vi "Sleep.vi"(8 "error in (no error)":errorcluster, 11 "CIFCorePlugin in":refnum<class "CIFCorePlugin.lvclass">) -> (0 "error out":errorcluster, 2 "Housekeep only":bool, 3 "CIFCorePlugin out":refnum<class "CIFCorePlugin.lvclass">)   [LabVIEW 2021, in "CIFCorePlugin.lvclass"]
uses:
  CIFCorePlugin.lvclass
  CIFCorePlugin.lvclass/CIFCorePlugin.ctl
  Common/Typedef/Errors.ctl
  Accessors/Read Sleep Limits (ns).vi
  Accessors/Timestamps/Write Target Wake TS.vi
  Accessors/Timestamps/Read Running TS.vi
  Accessors/Read Running Internal Data.vi
  Accessors/Read Timing Override.vi
  Accessors/Read Common Config.vi
  <vilib>/CIF Foundation/CIF Utilities/Errors/Append Error Location.vi
  <vilib>/CIF Foundation/CIF Utilities/Time/System Time/LabVIEW Time to TAI Time.vi
  Common/CIFCoreCommon.lvlib
  <vilib>/CIF Foundation/CIF Utilities/Time/Time_CIF_U.lvlib
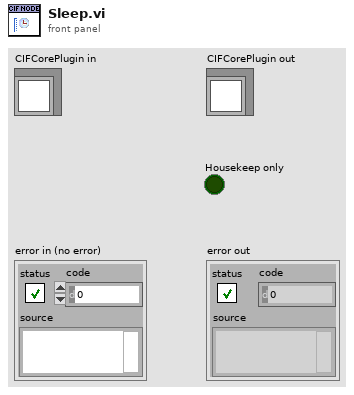
[diagram p1: front panel]
types:
  T1 = typedef "CIFCoreCommon.lvlib/Errors.ctl" = enum16{"Invalid Clock ID", "Long Sleep", "gRPC Server Not Found", "Config Parse", "Timestamp Wrap", "Delayed Execution", "Duplicate Channel", "Missing Channel", "Incorrect Type", "Flatten Error", "Unflatten Data", "Unique Name", "Plugin Not Found", "Plugin Type Not Found", "Plugin Version Not Found", "Manager Not Found", "Numerical Issue", "Time Jump", "Clock ID Match", "Channel Length", "Plugin Connection", "gRPC Server Connection", "PPL Name Match", "Build", "Config Log Parse", "Plugin Load"}
  T2 = typedef "CIFCoreCommon.lvlib/Timing Overrides.ctl" = cluster{"Override Timing":bool, "Skip Sleep":bool, "Period (s)":dbl}
  T3 = typedef "CIFCorePlugin.lvclass/Running Internal Data.ctl" = cluster{"Refresh":bool, "Iterations":i64, "Housekeep only":bool, "Configured period (ns)":i64, "Update channel OOB":bool}
  T4 = typedef "CIFCoreCommon.lvlib/Common Plugin Configuration.ctl" = cluster{"Period (s)":dbl, "Offset (us)":i32, "ClockID":u8, "Priority":i32, "Processor":i32}
  T5 = typedef "Time_CIF_U.lvlib/Future Time Event Limits.ctl" = cluster{"Maximum":i64, "Minimum":i64}
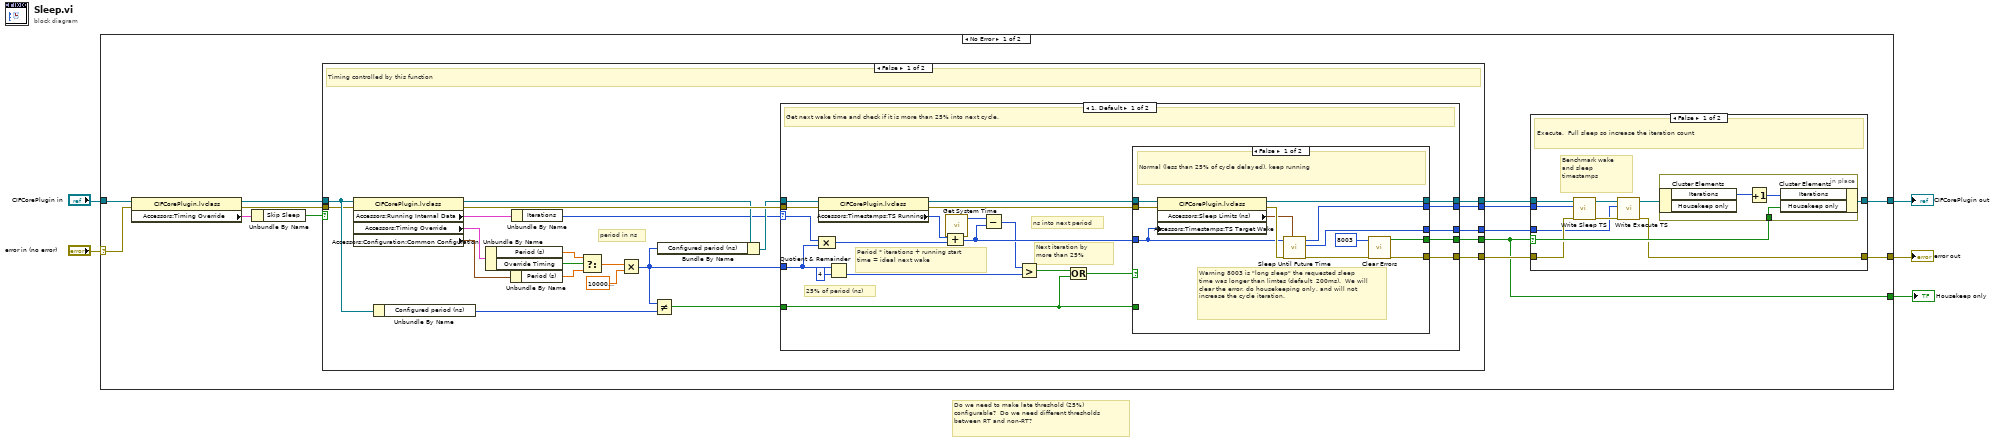
[diagram p0: block diagram]
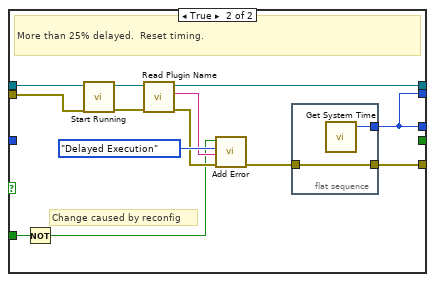
[diagram p2: hidden frame]
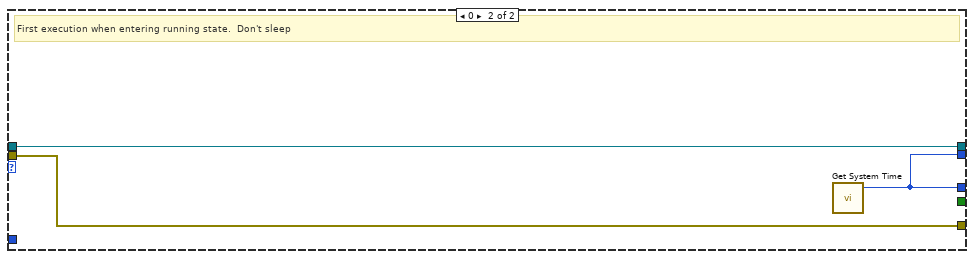
[diagram p3: hidden frame]
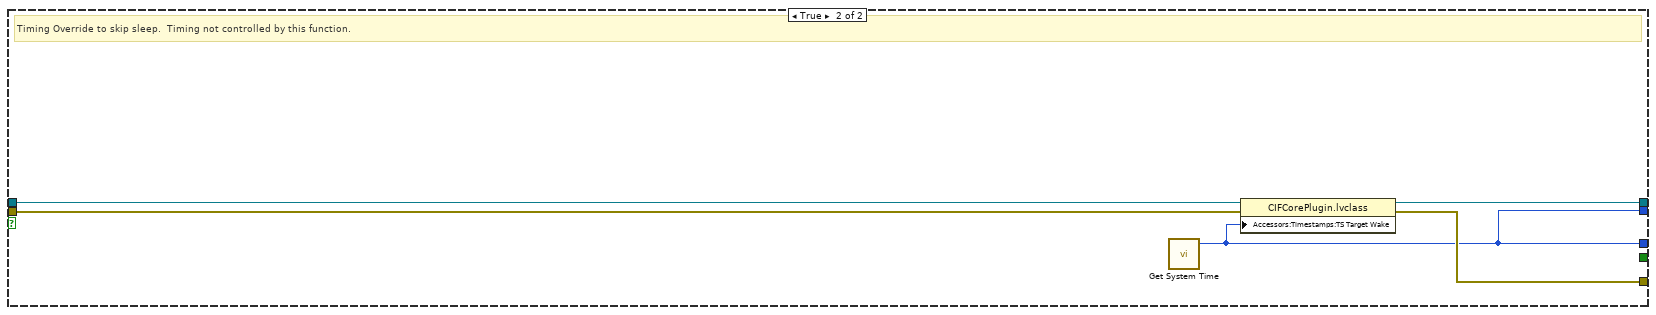
[diagram p4: hidden frame]
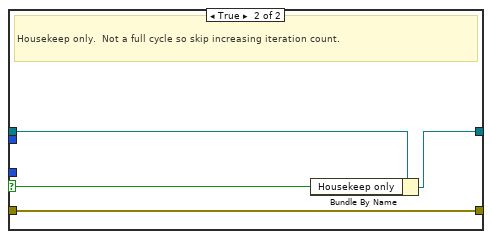
[diagram p5: hidden frame]
diagram:
  # "Do we need to make late threshold (25%) configurable?  Do we need different thresholds between RT and non-RT?"
  n1 = case shown="No Error" "error in (no error)" {
    selector: "error in (no error)" -> [w12 w115]
    tunnel: [w14 w115] -> w1
    tunnel: [w17 w114] -> w3
    tunnel: "CIFCorePlugin in" -> [w13 w114]
    tunnel: [w6 _] -> w2
    frame No Error {
      n2 = property class="CIFCorePlugin.lvclass"(reference=w13, error in=w12) -> (reference out=w11:refnum<class "CIFCorePlugin.lvclass">, error out=w10:errorcluster, "Accessors:Timing Override"=w9:T2)
      n3 = Unbundle By Name(w9) -> ("Skip Sleep"=w8:bool)
      n4 = case shown="False" w8 {
        tunnel: [w40 w95] -> w18
        tunnel: [w26 _] -> w6
        tunnel: [w23 w92] -> w16
        tunnel: [w22 w93] -> w15
        tunnel: w11 -> [w21 w96]
        tunnel: w10 -> [w20 w94]
        tunnel: [w19 w92] -> w7
        frame False {
          # "period in ns"
          # "Timing controlled by this function"
          n5 = property class="CIFCorePlugin.lvclass"(reference=w21, error in=w20) -> (reference out=w29:refnum<class "CIFCorePlugin.lvclass">, error out=w39:errorcluster, "Accessors:Running Internal Data"=w25:T3, "Accessors:Timing Override"=w31:T2, "Accessors:Configuration:Common Configuration"=w34:T4)
          n6 = Unbundle By Name(w21) -> ("Configured period (ns)"=w30:i64)
          n7 = Unbundle By Name(w31) -> ("Period (s)"=w33:dbl, "Override Timing"=w35:bool)
          n8 = Unbundle By Name(w34) -> ("Period (s)"=w38:dbl)
          n9 = Unbundle By Name(w25) -> ("Iterations"=w24:i64)
          n10 = Select(t=w33, s=w35, f=w38) -> (s? t:f=w36:dbl)
          n11 = Multiply(x=w36, y=1000000000.0 ("x")) -> (x*y=w27:i64)
          n12 = Not Equal?(x=w27, y=w30) -> (x != y?=w32:bool)
          n13 = Bundle By Name(cluster=w29, "Configured period (ns)"=w27) -> (w28:refnum<class "CIFCorePlugin.lvclass">)
          n14 = case shown="1, Default" w24 {
            selector: w24 -> [w45 _]
            tunnel: [w60 w91] -> w40
            tunnel: w39 -> [w61 w90]
            tunnel: w28 -> [w52 w91]
            tunnel: [w59 w90] -> w22
            tunnel: w27 -> [w42 _]
            tunnel: w32 -> [w56 _]
            tunnel: [w55 _] -> w26
            tunnel: [w54 w89] -> w23
            tunnel: [w53 w89] -> w19
            frame 1, Default {
              # "ns into next period"
              # "25% of period (ns)"
              # "Next iteration by more than 25%"
              # "Period * iterations + running start time = ideal next wake"
              # "Get next wake time and check if it is more than 25% into next cycle."
              n15 = property class="CIFCorePlugin.lvclass"(reference=w52, error in=w61) -> (reference out=w41:refnum<class "CIFCorePlugin.lvclass">, error out=w58:errorcluster, "Accessors:Timestamps:TS Running"=w51:i64)
              n16 = Compound Arithmetic op=MULTIPLY(w45, w42) -> (w50:i64)
              n17 = Quotient & Remainder(x=w42, y=i64 4) -> (floor(x/y)=w43:i64)  [unwired: 1 out]
              n18 = call <vilib>:"Get System Time.vi"() -> ("Time (ns)"=w49:i64)  [unwired: 5 in]
              n19 = Compound Arithmetic op=ADD(w51, w50) -> (w48:i64)
              n20 = Subtract(x=w49, y=w48) -> (x-y=w44:i64)
              n21 = Greater?(x=w44, y=w43) -> (0:w47:bool)
              n22 = Compound Arithmetic op=OR(w47, w56) -> (w57:bool)
              n23 = case shown="False" w57 {
                tunnel: w41 -> [w64 w86]
                tunnel: [w62 w81] -> w60
                tunnel: w58 -> [w73 w85]
                tunnel: [w72 w74] -> w59
                tunnel: w56 -> [_ w78]
                tunnel: w48 -> [w67 _]
                tunnel: [w70 _] -> w55
                tunnel: [w65 w76] -> w54
                tunnel: [w66 w76] -> w53
                frame False {
                  # "Warning 8003 is \"long sleep\" the requested sleep time was longer than limtes (default  200ms).  We will clear the error, do housekeeping only, and will not increase the cycle iteration."
                  # "Normal (less than 25% of cycle delayed), keep running"
                  n24 = property class="CIFCorePlugin.lvclass"(reference=w64, error in=w73, "Accessors:Timestamps:TS Target Wake"=w67) -> (reference out=w62:refnum<class "CIFCorePlugin.lvclass">, error out=w69:errorcluster, "Accessors:Sleep Limits (ns)"=w63:T5)
                  n25 = call <vilib>:"Sleep Until Future Time.vi"("FTE Limits (ns)"=w63, "error in (no error)"=w69, "Wake Time (ns)"=w67) -> ("error out"=w68:errorcluster, "Wake Time (ns)"=w65:i64, "Sleep TIme"=w66:i64)  [unwired: 6 in]
                  n26 = call <vilib>:"Clear Errors.vi"("error in (no error)"=w68, "specific error code to clear (0: all)"=8003 ("code")) -> ("error out"=w72:errorcluster, "specific error cleared?"=w70:bool)  [unwired: 4 in]
                }
                frame True {
                  # "Change caused by reconfig"
                  # "More than 25% delayed.  Reset timing."
                  n27 = Not(x=w78) -> (.not. x?=w77:bool)
                  n28 = call "Start Running.vi"("error in (no error)"=w85, "CIFCorePlugin in"=w86) -> ("error out"=w79:errorcluster, "CIFCorePlugin out"=w80:refnum<class "CIFCorePlugin.lvclass">)  [unwired: 8 in]
                  n29 = call "Read Plugin Name.vi"("error in (no error)"=w79, "CIFTemplateNode in"=w80) -> ("error out"=w82:errorcluster, "Plugin Name"=w83:string, "CIFTemplateNode out"=w81:refnum<class "CIFCorePlugin.lvclass">)  [unwired: 7 in]
                  n30 = call <vilib>:"Add Error.vi"("error in (no error)"=w82, "String to Append"=w83, "Error"=Errors."Delayed Execution", "Insert Error"=w77) -> ("error out"=w75:errorcluster)  [unwired: 7 in]
                  n31 = flat-sequence {
                    tunnel: [w88] -> w76
                    tunnel: w75 -> [w87]
                    tunnel: [w87] -> w74
                    frame #0 {
                      n32 = call <vilib>:"Get System Time.vi"() -> ("Time (ns)"=w88:i64)  [unwired: 5 in]
                    }
                  }
                }
              }
            }
            frame 0 {
              # "First execution when entering running state.  Don't sleep"
              n33 = call <vilib>:"Get System Time.vi"() -> ("Time (ns)"=w89:i64)  [unwired: 5 in]
            }
          }
        }
        frame True {
          # "Timing Override to skip sleep.  Timing not controlled by this function."
          n34 = call <vilib>:"Get System Time.vi"() -> ("Time (ns)"=w92:i64)  [unwired: 5 in]
          n35 = property class="CIFCorePlugin.lvclass"(reference=w96, error in=w94, "Accessors:Timestamps:TS Target Wake"=w92) -> (reference out=w95:refnum<class "CIFCorePlugin.lvclass">, error out=w93:errorcluster)
        }
      }
      n36 = case shown="False" w6 {
        selector: w6 -> [w105 w111]
        tunnel: w18 -> [w99 w113]
        tunnel: [w106 w112] -> w17
        tunnel: w16 -> [w98 _]
        tunnel: w15 -> [w101 w110]
        tunnel: [w103 w110] -> w14
        tunnel: w7 -> [w100 _]
        frame False {
          # "Benchmark wake and sleep timestamps"
          # "Execute.  Full sleep so increase the iteration count"
          n37 = call "Write Sleep TS.vi"("error in (no error)"=w101, "Sleep"=w100, "CIFCorePlugin in"=w99) -> ("error out"=w102:errorcluster, "CIFCorePlugin out"=w97:refnum<class "CIFCorePlugin.lvclass">)  [unwired: 7 in]
          n38 = call "Write Execute TS.vi"("error in (no error)"=w102, "Execute"=w98, "CIFCorePlugin in"=w97) -> ("error out"=w103:errorcluster, "CIFCorePlugin out"=w104:refnum<class "CIFCorePlugin.lvclass">)  [unwired: 7 in]
          n39 = in-place {
            in-place-border: w105 -> [w107]
            n40 = in-place-cluster #1(w104) -> ("Iterations"=w108:i64)  [unwired: 1 out]
            n41 = Increment(x=w108) -> (x+1=w109:i64)
            n42 = in-place-cluster #1("Iterations"=w109, "Housekeep only"=w107) -> (w106:refnum<class "CIFCorePlugin.lvclass">)
          }
        }
        frame True {
          # "Housekeep only.  Not a full cycle so skip increasing iteration count."
          n43 = Bundle By Name(cluster=w113, "Housekeep only"=w111) -> (w112:refnum<class "CIFCorePlugin.lvclass">)
        }
      }
    }
    frame Error {
    }
  }
  "error out" <- w1
  "CIFCorePlugin out" <- w3
  "Housekeep only" <- w2
